vi "CN0d.vi"(1 "Downlink Free Space path Loss  (dB)":dbl, 2 "G/T ground (dBK-1)":dbl, 3 "EIRP sat (dBW)":dbl) -> (0 "C/N0d (dBHz)":dbl)   [LabVIEW 2015]
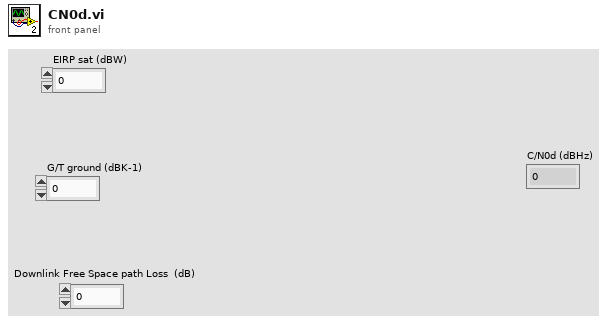
[diagram p1: front panel]
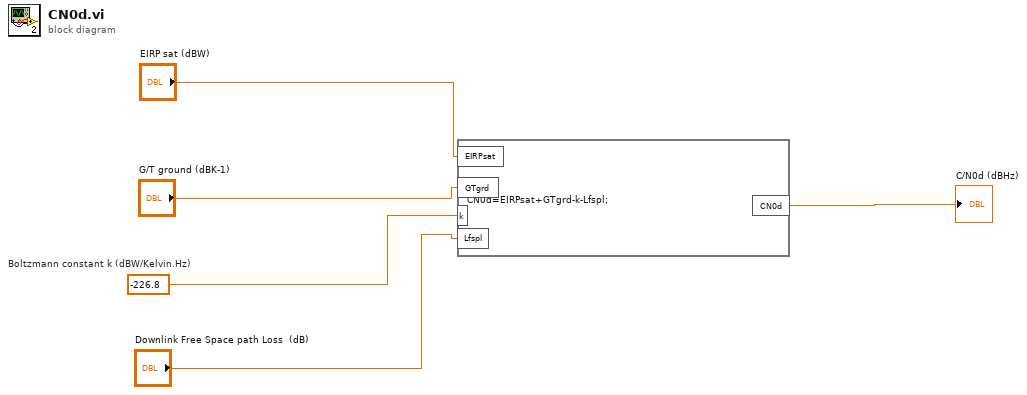
[diagram p0: block diagram]
diagram:
  w3 = -226.8  # Boltzmann constant k (dBW/Kelvin.Hz)
  n1 = formula code="CN0d=EIRPsat+GTgrd-k-Lfspl;"("EIRPsat"="EIRP sat (dBW)", "GTgrd"="G/T ground (dBK-1)", "k"=w3, "Lfspl"="Downlink Free Space path Loss  (dB)") -> ("CN0d"=→"C/N0d (dBHz)":dbl)
